vi "WILT Read General Configuration.vi"(0 "File Path Input":T1[](array[typedef]), 5 "Error In":errorcluster) -> (6 "Scan Rate":dbl, 8 "Save Rate":dbl, 10 "Current Threshold":dbl, 12 "Send Restart Every? (Sec)":dbl, 14 "State Machine String":string, 15 "File Path Output":T1[](array[typedef]), 16 "Station Timeout Values (1-56) Seconds":dbl[](array[numeric]), 17 "Drying Time (Min)":dbl[](array[numeric]), 19 "Error Out":errorcluster)   [LabVIEW 2016]
uses:
  Utility/Save File/File Setup (Public)/Type Definition/Save File DOE File Path Control.ctl
  Utility/Save File/File Setup (Public)/Type Definition/Save File DOE Data Save Filepaths.ctl
  Utility/Type Definitions/UTILITY Default File Create.ctl
  <vilib>/Utility/file.llb/Read Delimited Spreadsheet (string).vi
  Utility/Save File/Save File.lvlib
  Utility/Save File/File Setup.lvlib
panel:
  out "Station Timeout Values":string
  in  "General Configuration (Debug ONLY)":path=path "C:/Users/220038920/Desktop/Project/NI-2010/Trunk/Dryer Wilt/Documentation/General Configuration.txt"
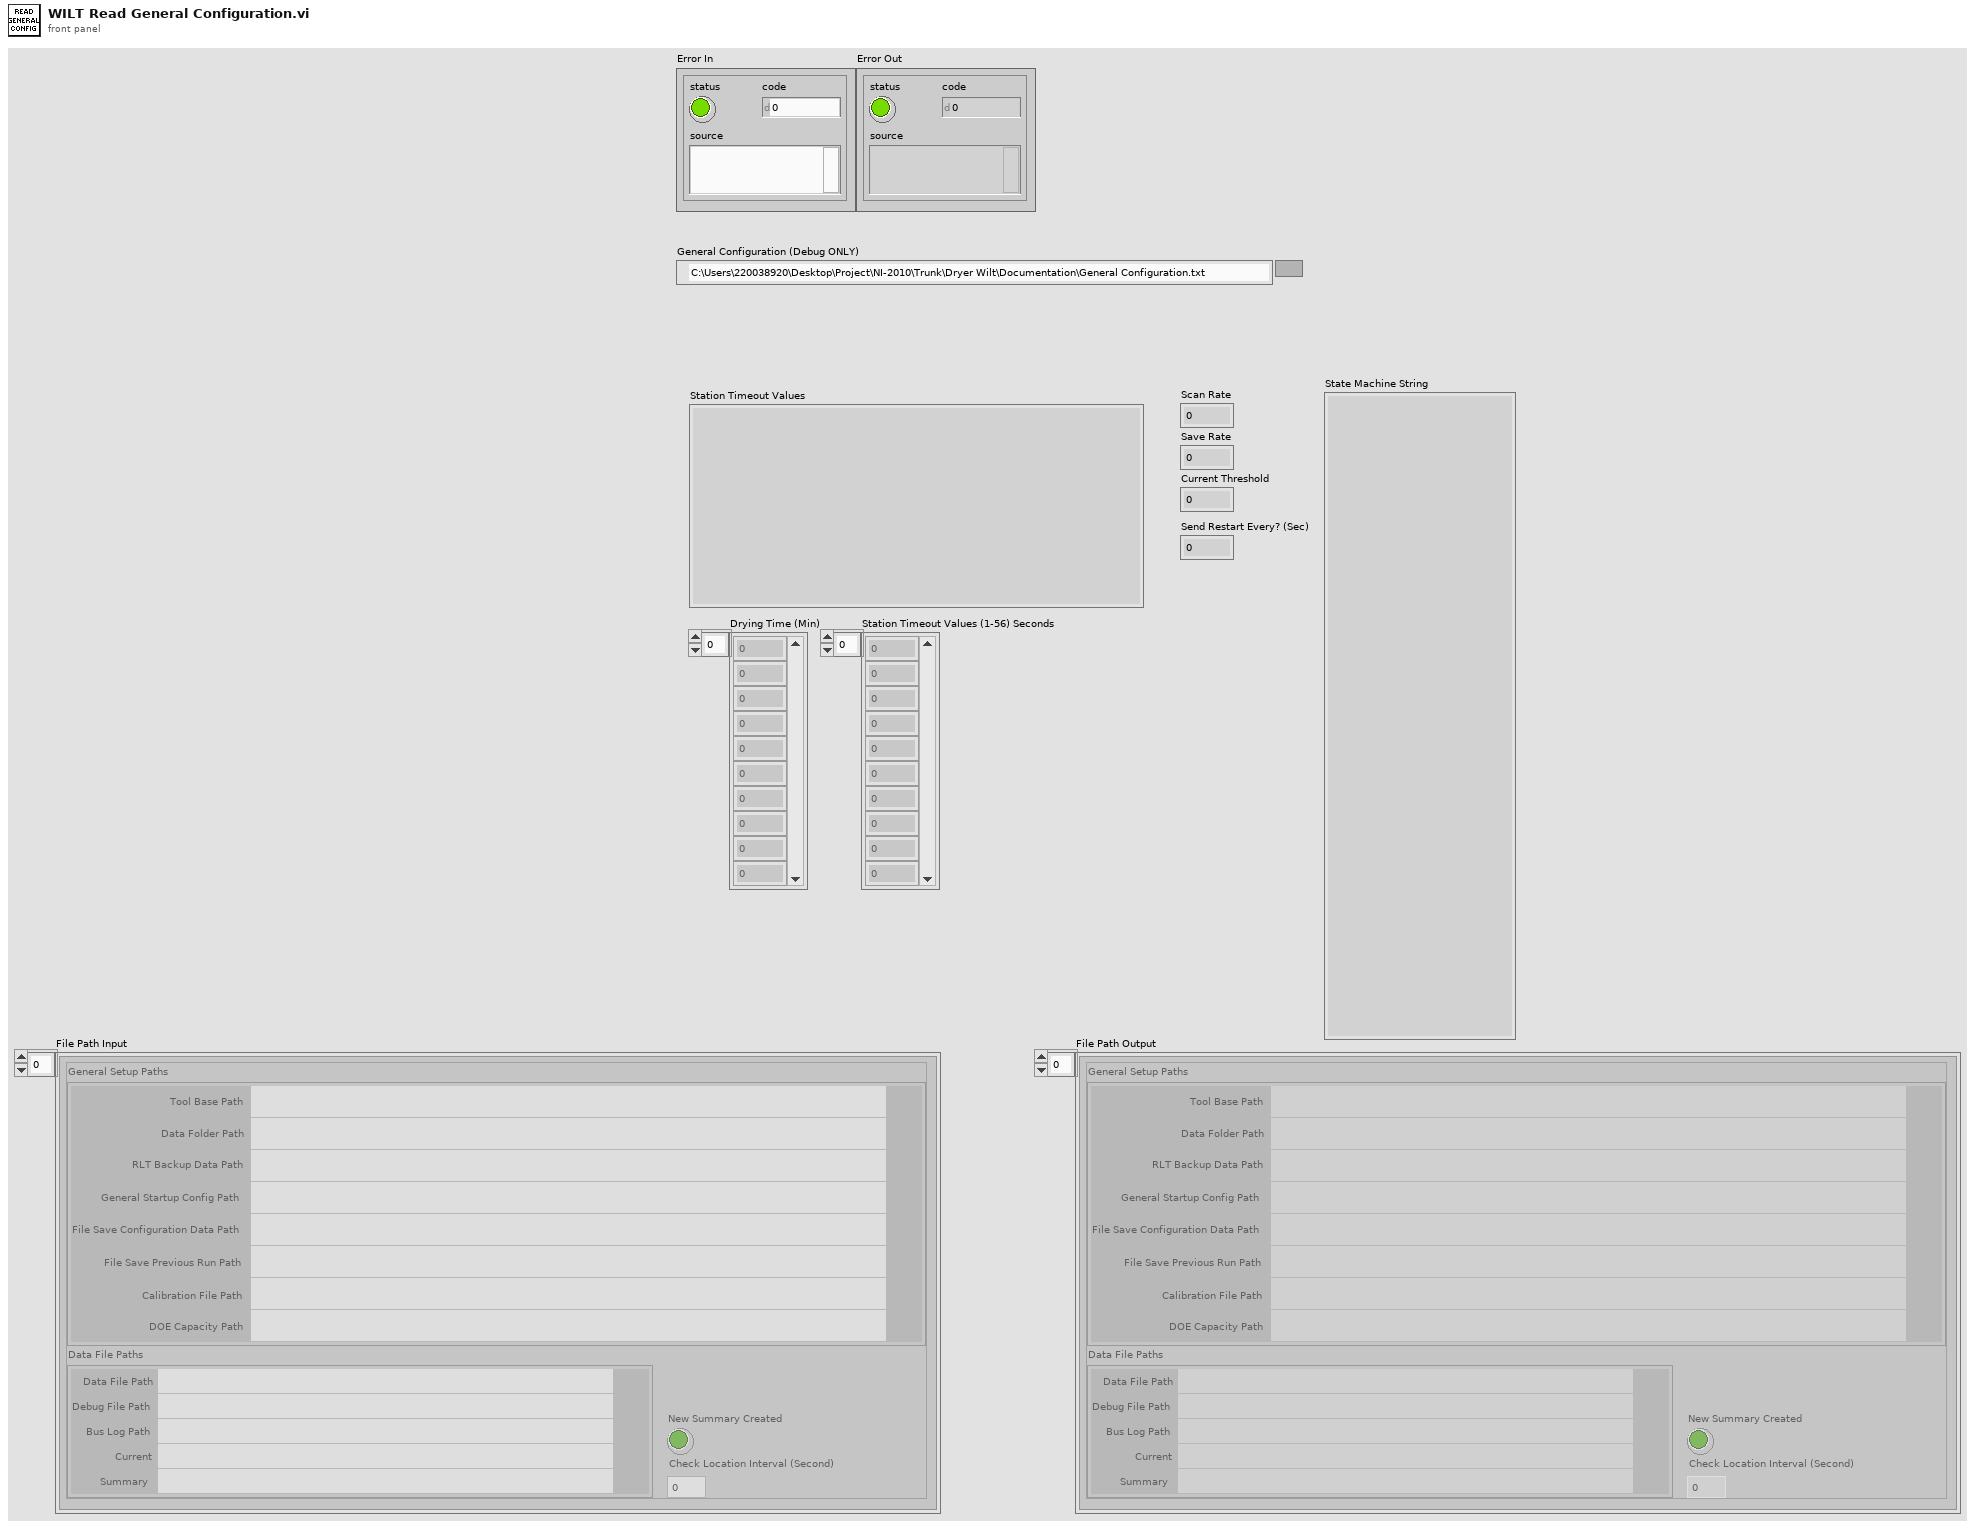
[diagram p1: front panel]
types:
  T1 = typedef "File Setup.lvlib/Save File DOE File Path Control.ctl" = cluster{"General Setup Paths":cluster{"Calibration File Path":path, "DOE Capacity Path":path, "Data Folder Path":path, "RLT Backup Data Path":path, "Tool Base Path":path, "General Startup Config Path":path, "File Save Previous Run Path":path, "File Save Configuration Data Path":path}, "Data File Paths":T2, "New Summary Created":bool, "Check Location Interval (Second)":i32}
  T2 = typedef "File Setup.lvlib/Save File DOE Data Save Filepaths.ctl" = cluster{"Data File Path":path, "Debug File Path":path, "Bus Log Path":path, "Current":path, "Summary":path}
  T3 = typedef "UTILITY Default File Create.ctl" = enum16{"Configuration File", "Debug Search File", "WILT Water Injection Times", "WILT Agilent Assignment", "WILT Save Status Path", "WILT General Config"}
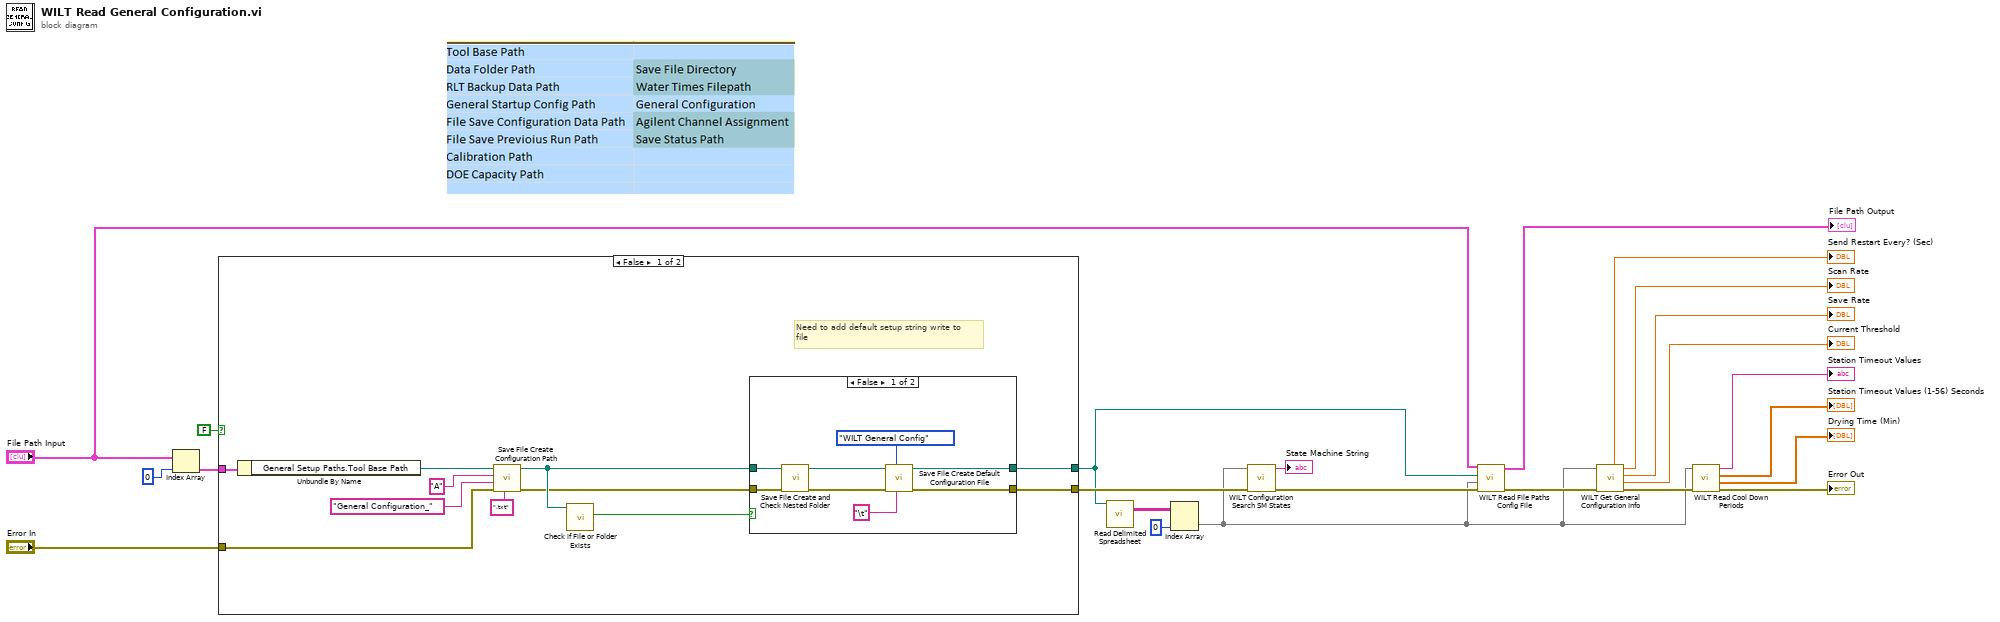
[diagram p0: block diagram]
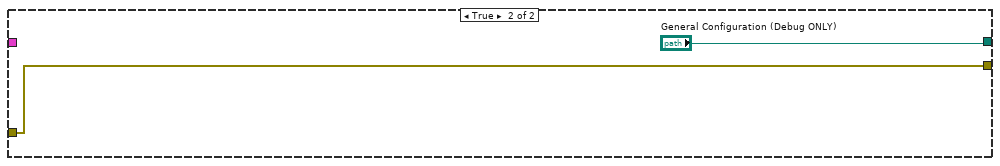
[diagram p3: hidden frame]
diagram:
  n1 = Index Array(array="File Path Input", index=0) -> (element=w6:T1)
  n2 = case shown="False" FALSE {
    tunnel: [w27 "General Configuration (Debug ONLY)"] -> w2
    tunnel: w6 -> [w26 _]
    tunnel: [w25 w45] -> w9
    tunnel: "Error In" -> [w24 w45]
    frame False {
      # "Need to add default setup string write to\nfile"
      n3 = Unbundle By Name(w26) -> ("General Setup Paths.Tool Base Path"=w34:path)
      n4 = call "Save File Create Configuration Path.vi"("File Type (.ini)"=".txt", "Error In"=w24, "Configuration Name"="General Configuration_", "Station ID"="A", "Tool Base Path"=w34) -> ("Error Out"=w28:errorcluster, "New Configuration File Path"=w29:path)  [unwired: 5 in]
      n5 = call <vilib>:"Check if File or Folder Exists.vi"("path"=w29) -> ("file or folder exists?"=w30:bool)  [unwired: 8 in, 2 out]
      n6 = case shown="False" w30 {
        tunnel: w29 -> [w42 w44]
        tunnel: [w38 w44] -> w27
        tunnel: w28 -> [w41 w43]
        tunnel: [w39 w43] -> w25
        frame False {
          n7 = call "Save File Create and Check Nested Folder.vi"("error in (no error)"=w41, "Extracted File Name"=w42) -> ("error out"=w40:errorcluster, "File Path"=w37:path)  [unwired: 7 in, 1 out]
          n8 = call "Save File Create Default Configuration File.vi"("delimiter (\\t)"="\t" ("delimiter (\\t)"), "Default File Create"=UTILITY_Default_File_Create."WILT General Config", "Error In"=w40, "File Path In"=w37) -> ("Error Out"=w39:errorcluster, "File Path Out"=w38:path)  [unwired: 6 in]
        }
        frame True {
        }
      }
    }
    frame True {
    }
  }
  n9 = call-poly <vilib>:"Read Delimited Spreadsheet.vi"("file path (dialog if empty)"=w2) -> ("all rows"=w1:string[][])  [unwired: 9 in, 5 out]
  n10 = Index Array(array=w1, index (col)=0 ("disabled index (col)")) -> (element=w3:string[])  [unwired: 1 in]
  n11 = call "WILT Configuration Search SM States.vi"("Error In"=w9, "Full Data States"=w3) -> ("Error Out"=w17:errorcluster, "SM String"=→"State Machine String":string)  [unwired: 8 in]
  n12 = call "WILT Read File Paths Config File.vi"("Error In"=w17, "Config Data Input"=w3, "General Configuration File Path"=w2, "File Path Input"="File Path Input") -> ("Error Out"=w12:errorcluster, "File Path Output"=→"File Path Output":T1[])  [unwired: 6 in]
  n13 = call "WILT Get General Configuration Info.vi"("Error In"=w12, "all rows"=w3) -> ("Error Out"=w11:errorcluster, "Current Threshold"=→"Current Threshold":dbl, "Save Rate"=→"Save Rate":dbl, "Scan Rate"=→"Scan Rate":dbl, "Send Restart Every? (Sec)"=→"Send Restart Every? (Sec)":dbl)  [unwired: 5 in]
  n14 = call "WILT Read Cool Down Periods.vi"("Error In"=w11, "Input Cool Down Data"=w3) -> ("Error Out"=→"Error Out":errorcluster, "Drying Time (Min)"=→"Drying Time (Min)":dbl[], "Station Timeout Values (1-56) Seconds"=→"Station Timeout Values (1-56) Seconds":dbl[], "Station Timeout Values"=→"Station Timeout Values":string)  [unwired: 6 in]
